vi "Paint Button on Mouse Over.vi"(7 "New Active Button":i32, 8 "error in (no error)":errorcluster, 9 "Array in":refnum<vi>, 10 "Tip String Ref":refnum<vi>, 11 "Button States in":refnum<class "Button.lvclass">[](array[class])) -> (0 "error out":errorcluster, 3 "Button States out":refnum<class "Button.lvclass">[](array[class]))   [LabVIEW 2012, in "Toolbar.xctl"]
uses:
  Toolbar.xctl
  Button_Class/Button.lvclass
  Button_Class/Type Defs/Button Status.ctl
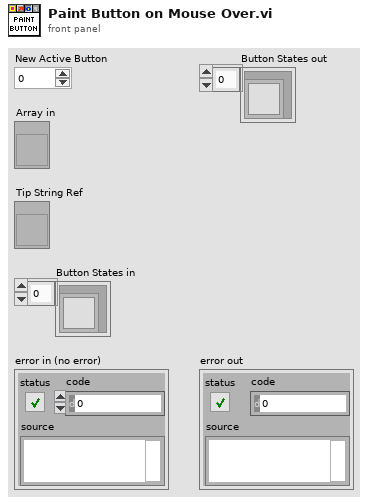
[diagram p1: front panel]
types:
  T1 = typedef "Button.lvclass/Button Status.ctl" = enum16{"Off", "Hover", "On", "Disabled"}
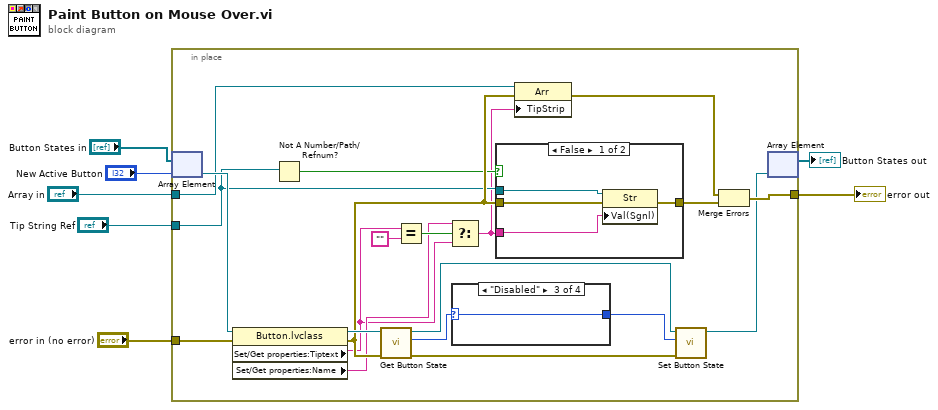
[diagram p0: block diagram]
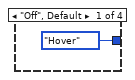
[diagram p3: hidden frame]
diagram:
  n1 = in-place {
    in-place-border: "error in (no error)" -> [w21]
    in-place-border: [w16] -> w6
    in-place-border: "Tip String Ref" -> [w15]
    in-place-border: "Array in" -> [w14]
    n2 = in-place-array #1("Button States in", "New Active Button") -> (w27:refnum<class "Button.lvclass">)
    n3 = property class="Button.lvclass"(reference=w27, error in=w21) -> (reference out=w22:refnum<class "Button.lvclass">, error out=w20:errorcluster, "Set/Get properties:Tiptext"=w9:string, "Set/Get properties:Name"=w10:string)
    n4 = Not A Number/Path/Refnum?(number/path/refnum=w15) -> (NaN/Path/Refnum?=w19:bool)
    n5 = call-dynamic "Get Button State.vi"("error in (no error)"=w20, "Button in"=w22) -> ("error out"=w23:errorcluster, "State"=w25:T1, "Button out"=w26:refnum<class "Button.lvclass">)  [unwired: 1 in, 6 out]
    n6 = Equal?(x=w9, y="") -> (x = y?=w11:bool)
    n7 = Select(t=w10, s=w11, f=w9) -> (s? t:f=w8:string)
    n8 = case shown="\"Disabled\"" w25 {
      selector: w25 -> [_ w34 w35 w36]
      tunnel: [Button_Status."Hover" ("State") w34 w35 w36] -> w24
      frame "Off", Default {
      }
      frame "On" {
      }
      frame "Disabled" {
      }
      frame "Hover" {
      }
    }
    n9 = case shown="False" w19 {
      tunnel: w20 -> [w31 w32]
      tunnel: w8 -> [w30 _]
      tunnel: [w29 w32] -> w17
      tunnel: w15 -> [w28 _]
      frame False {
        n10 = property class="Str"(reference=w28, error in=w31, "Val(Sgnl)"=w30) -> (error out=w29:errorcluster)  [unwired: 1 out]
      }
      frame True {
      }
    }
    n11 = property on="Property Node" class="Arr"(reference=w14, error in=w20, "TipStrip"=w8) -> (error out=w18:errorcluster)  [unwired: 1 out]
    n12 = call-dynamic "Set Button State.vi"("error in (no error)"=w23, "State"=w24, "Button in"=w26) -> ("Button out"=w13:refnum<class "Button.lvclass">)  [unwired: 8 out]
    n13 = Merge Errors(w18, w17) -> (w16:errorcluster)
    n14 = in-place-array #1(w13) -> (→"Button States out":refnum<class "Button.lvclass">[])  [unwired: 1 out]
  }
  "error out" <- w6
